vi "String into array_0.vi"() -> ()   [LabVIEW 2015]
panel:
  in  "stop":bool
  in  "Tab Control":enum32{"Page 1"}(tab)
  in  "String":string
  out "Array":string[](array[string])
  out "length":i32
  # "Convert String into Array"
  # "Pardeep Kumar"
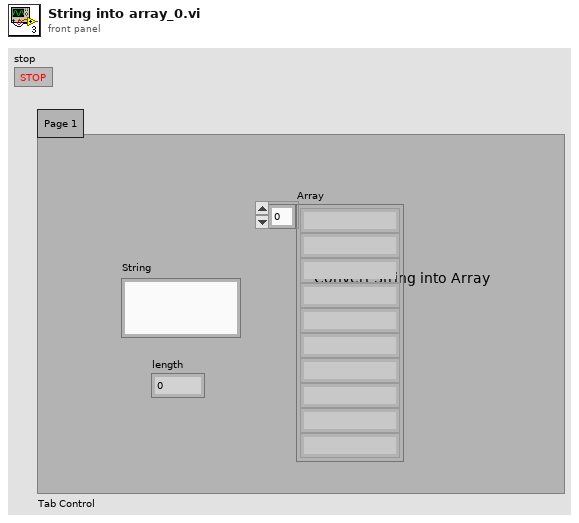
[diagram p1: front panel]
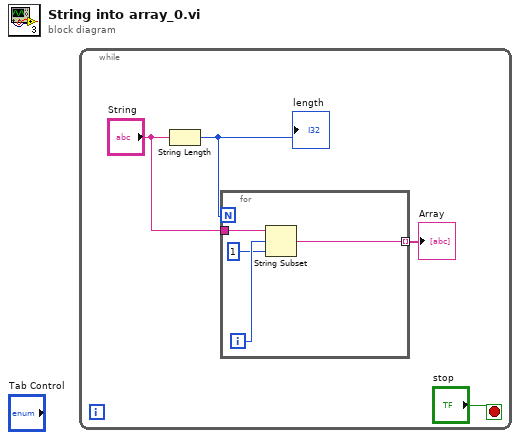
[diagram p0: block diagram]
diagram:
  n1 = while {
    stop <- "stop" stop-if-true
    n2 = String Length(string="String") -> (length=w4:i32)
    "length" <- w4
    n3 = for {
      N: w4 -> [_]
      tunnel: "String" -> [w8]
      tunnel: [w5] -> w2 mode=indexing
      i -> [w7]
      n4 = String Subset(string=w8, offset (0)=w7, length (rest)=1 ("length (rest)")) -> (substring=w5:string)
    }
    "Array" <- w2
  }
